vi "GetLimitAll.vi"(4 "StepError":errorcluster, 5 "坐标变换":dbl[](array[numeric]), 6 "PositionIn":i32[](array[numeric]), 7 "com in":refnum<visa-resource-name>) -> (0 "StepErrorOut":errorcluster, 2 "限位输出":bool[](array[boolean]), 3 "com out":refnum<visa-resource-name>)   [LabVIEW 2018]
uses:
  Device VIs/Verbal.vi
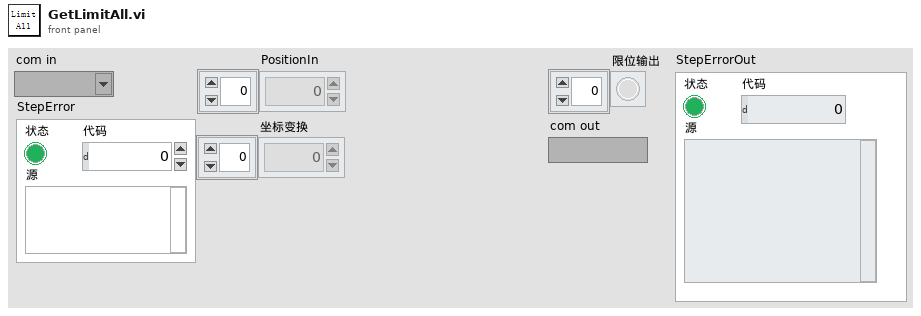
[diagram p1: front panel]
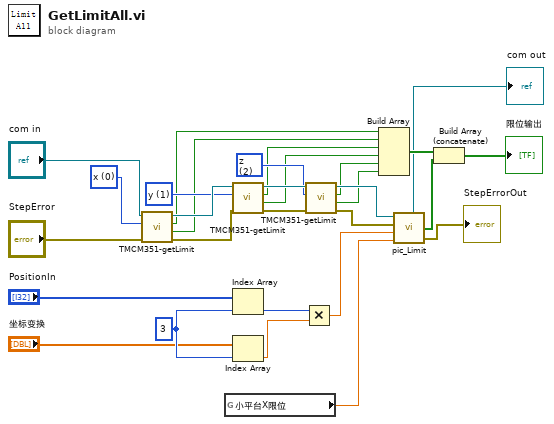
[diagram p0: block diagram]
diagram:
  w16 = 3 ("索引")
  w22 = u8 2 items=["x", "y", "z"] ("motor")
  w23 = u8 1 items=["x", "y", "z"] ("motor")
  w24 = u8 0 items=["x", "y", "z"] ("motor")
  n1 = call "TMCM351-getLimit.vi"("错误输入"="StepError", "motor"=w24, "com in"="com in") -> ("错误输出"=w28:errorcluster, "right limit"=w10:bool, "left limit"=w11:bool, "com out"=w29:refnum<visa-resource-name>)  [unwired: 1 in]
  n2 = global read "Verbal.vi" "小平台X限位"() -> (w18:dbl)
  n3 = call "TMCM351-getLimit.vi"("错误输入"=w28, "motor"=w23, "com in"=w29) -> ("错误输出"=w21:errorcluster, "right limit"=w8:bool, "left limit"=w9:bool, "com out"=w27:refnum<visa-resource-name>)  [unwired: 1 in]
  n4 = Index Array(array="PositionIn", index=w16) -> (element=w14:i32)
  n5 = Index Array(array="坐标变换", index=w16) -> (element=w13:dbl)
  n6 = Multiply(x=w14, y=w13) -> (x*y=w12:dbl)
  n7 = call "TMCM351-getLimit.vi"("错误输入"=w21, "motor"=w22, "com in"=w27) -> ("错误输出"=w19:errorcluster, "right limit"=w6:bool, "left limit"=w7:bool, "com out"=w20:refnum<visa-resource-name>)  [unwired: 1 in]
  n8 = Build Array(w11, w10, w9, w8, w7, w6) -> (w5:bool[])
  n9 = call "pic_Limit.vi"("小平台X轴限位"=w18, "小平台X轴当前位置"=w12, "错误输入"=w19, "com in"=w20) -> ("错误输出"=→"StepErrorOut":errorcluster, "Limit out"=w4:bool[], "com out"=→"com out":refnum<visa-resource-name>)
  n10 = Build Array (concatenate)(w5, w4) -> (→"限位输出":bool[])
